vi "3D_viewer.vi"() -> ()   [LabVIEW 2015]
uses:
  <vilib>/Utility/miscctls.llb/LVRGBAColorTypeDef.ctl
  <vilib>/Utility/miscctls.llb/LV3DPointTypeDef.ctl
  <vilib>/picture/3D Picture Control/Object/Create Object (name).vi
  G_ALL.vi
  G_SEN.vi
  <vilib>/picture/3D Picture Control/NI_3D Picture Control.lvlib
panel:
  in  "obs":bool
  in  "lane":bool
  in  "map":bool
  in  "y":dbl(slide)=-32.45749613601231 scale=-1000.0..1000.0
  in  "x":dbl(slide)=53.2687651331719 scale=-1000.0..1000.0
  in  "reset camera 2":bool
  out "Translation":cluster{"X":sgl, "Y":sgl, "Z":sgl}
  out "appended path":path
  in  "reset camera":bool
  out "car obs":refnum<vi>
  out "3D Picture":refnum<vi>(3d-picture)
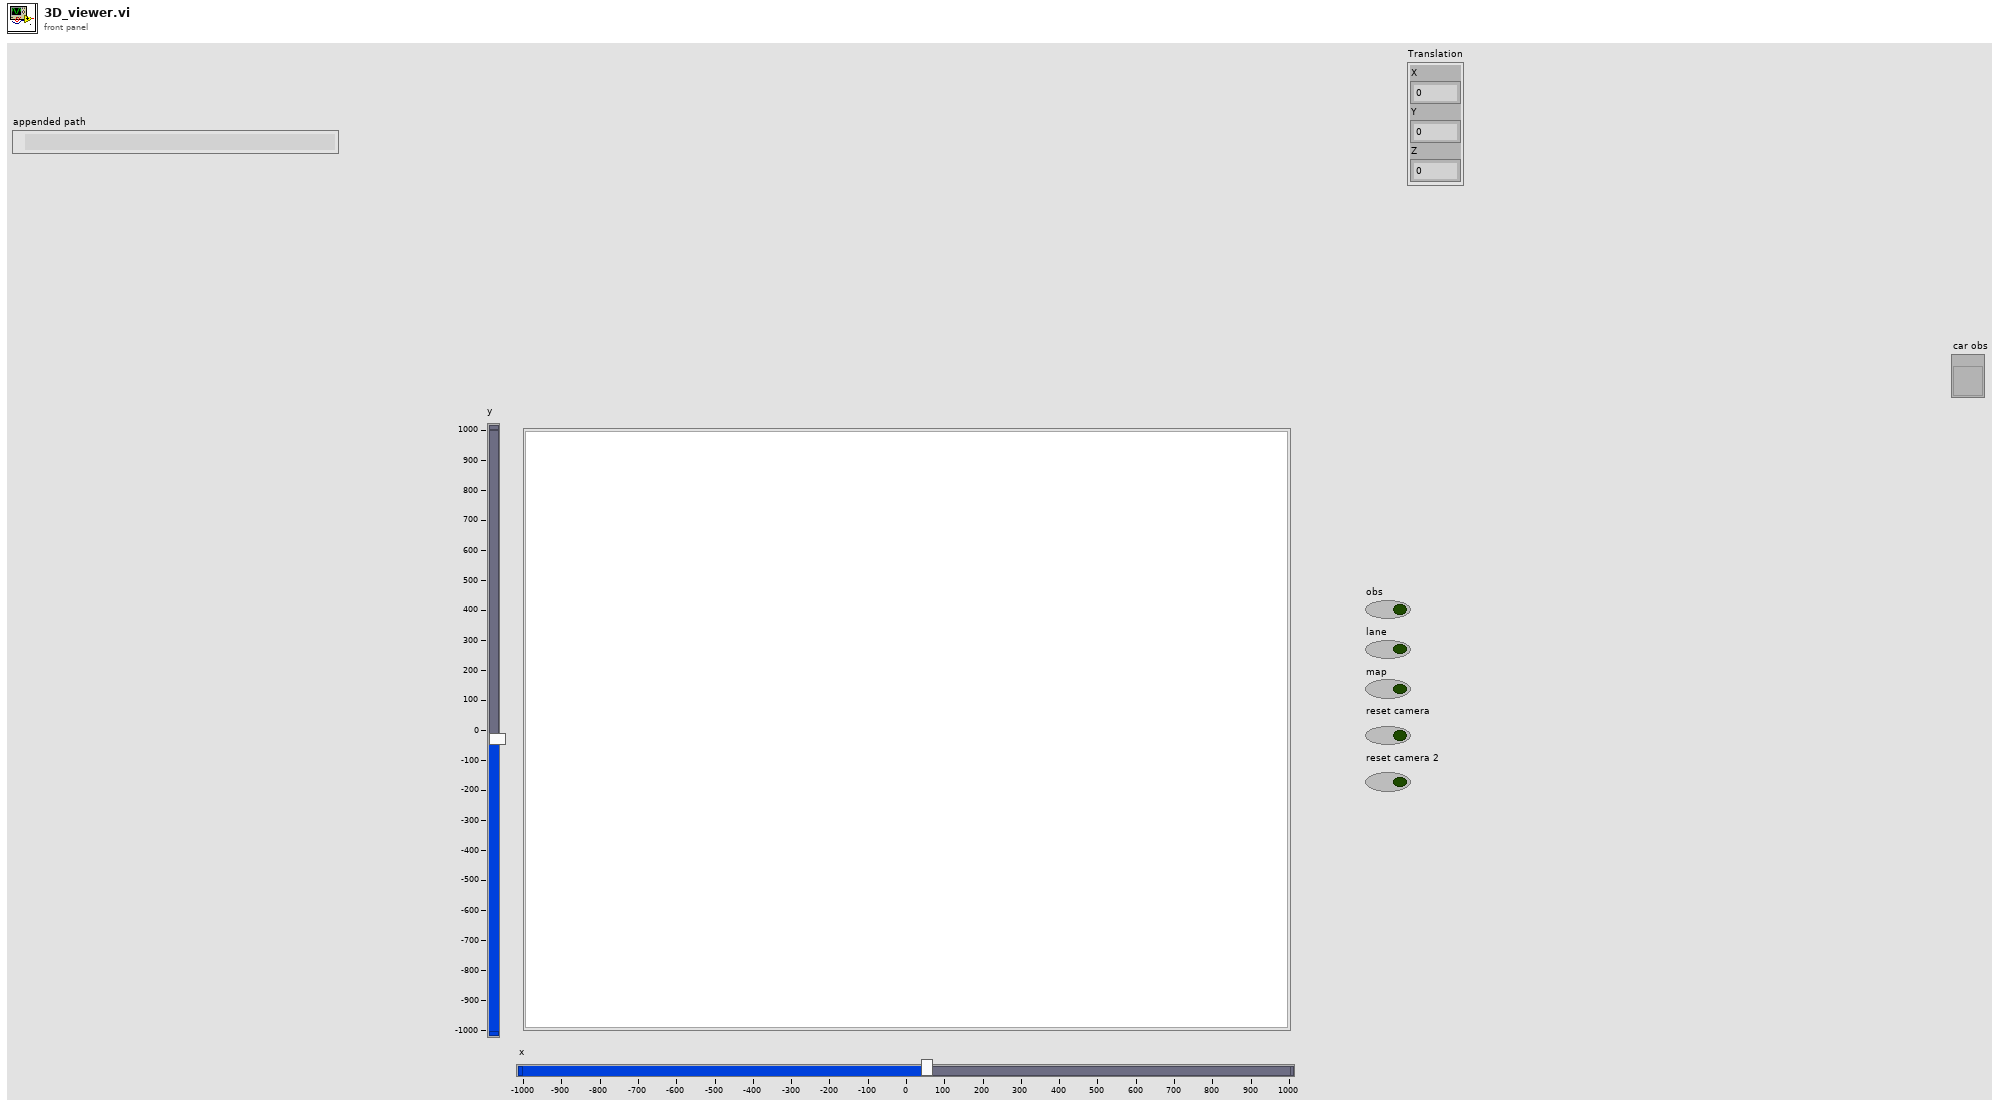
[diagram p1: front panel]
types:
  T1 = enum16{"None", "Spherical", "Flying", "Oriented"}
  T2 = cluster{"Red":sgl, "Green":sgl, "Blue":sgl, "Alpha":sgl}
  T3 = enum16{"Overall", "Per Primitive", "Per Vertex", "Binding Off"}
  T4 = typedef "LVRGBAColorTypeDef.ctl" = cluster{"Red":sgl, "Green":sgl, "Blue":sgl, "Alpha":sgl}
  T5 = enum16{"Points", "Lines", "Line Strip", "Line Loop", "Triangles", "Triangle Strip", "Triangle Fan", "Quads", "Quad Strip", "Polygon"}
  T6 = typedef "LV3DPointTypeDef.ctl" = cluster{"X":sgl, "Y":sgl, "Z":sgl}
  T7 = typedef "imagedata.ctl" = cluster{"image type":i32, "image depth":i32, "image":u8[], "mask":u8[], "colors":u32[], "Rectangle":cluster{"left":i16, "top":i16, "right":i16, "bottom":i16}}
  T8 = cluster{"left":i16, "top":i16, "right":i16, "bottom":i16}
  T9 = cluster{"left":sgl, "top":sgl, "right":sgl, "bottom":sgl}
  T10 = cluster{"Steer_input":dbl, "Steer_output":dbl, "VS_des":dbl, "VS_can":dbl, "heading":dbl, "auto":bool, "run":bool, "x":dbl, "y":dbl}
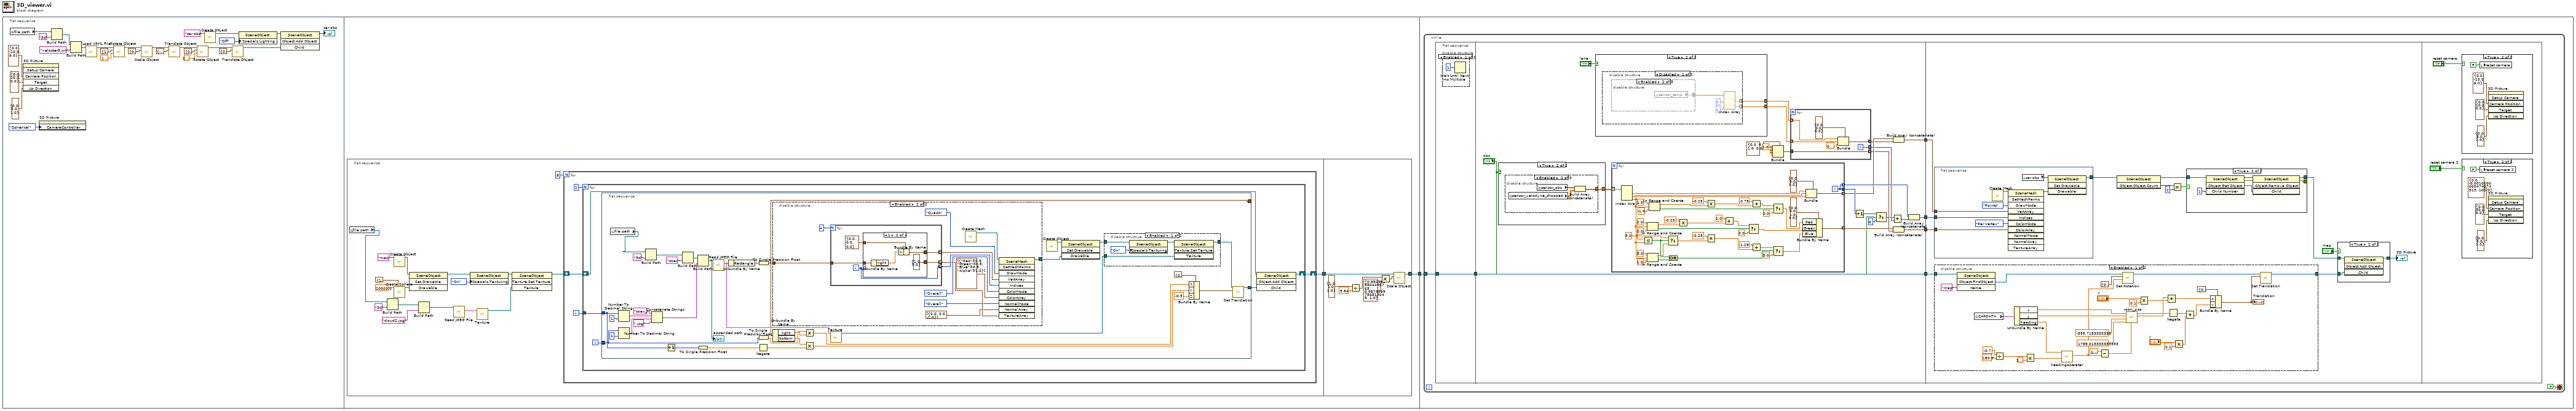
[diagram p0: block diagram]
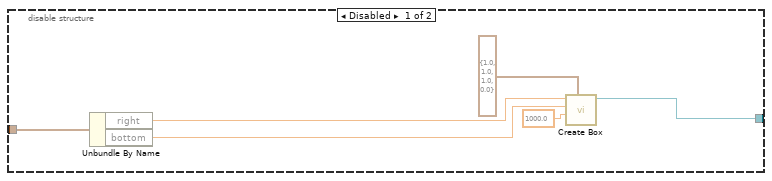
[diagram p3: hidden frame]
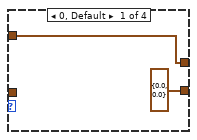
[diagram p4: hidden frame]
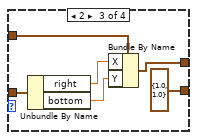
[diagram p5: hidden frame]
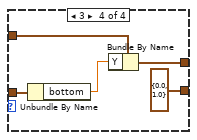
[diagram p6: hidden frame]
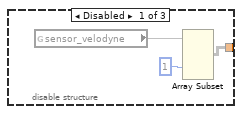
[diagram p9: hidden frame]
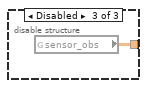
[diagram p10: hidden frame]
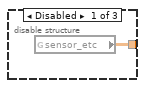
[diagram p12: hidden frame]
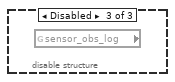
[diagram p13: hidden frame]
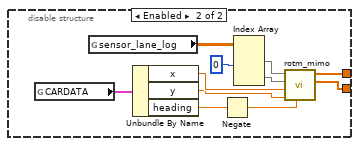
[diagram p14: hidden frame]
diagram:
  n1 = flat-sequence {
    tunnel: [w30] -> w1
    tunnel: w1 -> [w147]
    frame #0 {
      n2 = global read "G_ALL.vi" "file path"() -> (w2:path)
      n3 = invoke on="3D Picture" class="SceneGraphDisp (strict)" method="Setup Camera"("Camera Position"=cluster{"X":sgl, "Y":sgl, "Z":sgl} {"X"=0.0, "Y"=-10.0, "Z"=6.0}, "Target"=cluster{"X":sgl, "Y":sgl, "Z":sgl} {"X"=0.0, "Y"=10.0, "Z"=0.0}, "Up Direction"=cluster{"X":sgl, "Y":sgl, "Z":sgl} {"X"=0.0, "Y"=0.0, "Z"=1.0}) -> ()  [unwired: 3 in, 6 out]
      n4 = property on="3D Picture" class="SceneGraphDisp (strict)"("CameraController"=T1."Spherical" ("Camera Controller:Type")) -> ()  [unwired: 2 in, 2 out]
      n5 = Build Path(base path=w2, name or relative path="3d") -> (appended path=w25:path)
      n6 = Build Path(base path=w25, name or relative path="veloster3.wrl") -> (appended path=w27:path)
      n7 = call <vilib>:"Load VRML File.vi"("Path"=w27) -> ("Scene:Read Scene File"=w12:refnum<vi>)  [unwired: 9 in, 1 out]
      n8 = call <vilib>:"Rotate Object.vi"("Angle"=1.5707963267948966, "Axis"=cluster{"X":sgl, "Y":sgl, "Z":sgl} {"X"=1.0, "Y"=0.0, "Z"=0.0}, "Scene.Object In"=w12) -> ("Scene.Object Out"=w9:refnum<vi>)  [unwired: 7 in, 1 out]
      n9 = call <vilib>:"Scale Object.vi"("Scale"=cluster{"X":sgl, "Y":sgl, "Z":sgl} {"X"=0.055, "Y"=0.058, "Z"=0.058}, "Scene.Object In"=w9) -> ("Scene.Object Out"=w7:refnum<vi>)  [unwired: 8 in, 1 out]
      n10 = call <vilib>:"Translate Object.vi"("Translation"=cluster{"X":sgl, "Y":sgl, "Z":sgl} {"X"=-1.385, "Y"=-4.9, "Z"=-0.98}, "Scene.Object In"=w7) -> ("Scene.Object Out"=w15:refnum<vi>)  [unwired: 8 in, 1 out]
      n11 = call <vilib>:"Rotate Object.vi"("Angle"=3.141592653589793, "Axis"=cluster{"X":sgl, "Y":sgl, "Z":sgl} {"X"=0.0, "Y"=0.0, "Z"=1.0}, "Scene.Object In"=w15) -> ("Scene.Object Out"=w21:refnum<vi>)  [unwired: 7 in, 1 out]
      n12 = call-poly <vilib>:"Create Object.vi"("Name"="car obs") -> ("Scene:New Object"=w5:refnum<vi>)  [unwired: 9 in, 1 out]
      n13 = call <vilib>:"Translate Object.vi"("Translation"=cluster{"X":sgl, "Y":sgl, "Z":sgl} {"X"=0.0, "Y"=0.0, "Z"=0.2159}, "Scene.Object In"=w21) -> ("Scene.Object Out"=w22:refnum<vi>)  [unwired: 8 in, 1 out]
      n14 = property class="SceneObject"(reference=w5, "Specials.Lighting"=enum16{"Inherit Value", "Off", "On"}."Off" ("Specials:Lighting")) -> (reference out=w13:refnum<vi>)  [unwired: 1 in, 1 out]
      n15 = invoke class="SceneObject" method="Object.Add Object"(reference=w13, "Child"=w22) -> (reference out=→"car obs":refnum<vi>)  [unwired: 2 in, 3 out]
    }
    frame #1 {
      n16 = flat-sequence {
        tunnel: [w32] -> w29
        tunnel: [w145] -> w30
        tunnel: w29 -> [w146]
        frame #0 {
          n17 = global read "G_ALL.vi" "file path"() -> (w31:path)
          n18 = Build Path(base path=w31, name or relative path="3d") -> (appended path=w34:path)
          n19 = call-poly <vilib>:"Create Object.vi"("Name"="map") -> ("Scene:New Object"=w44:refnum<vi>)  [unwired: 9 in, 1 out]
          n20 = call <vilib>:"Create Sphere.vi"("Color"=T2 {"Red"=1.0, "Green"=1.0, "Blue"=1.0, "Alpha"=1.0}, "Radius"=sgl 20000.0) -> ("New Sphere Refnum"=w43:refnum<vi>)  [unwired: 8 in, 1 out]
          n21 = invoke class="SceneObject" method="Set Drawable"(reference=w44, "Drawable"=w43) -> (reference out=w42:refnum<vi>)  [unwired: 2 in, 3 out]
          n22 = Build Path(base path=w34, name or relative path="cloud2.jpg") -> (appended path=w33:path)
          n23 = call <vilib>:"Read JPEG File.vi"("path to JPEG file"=w33) -> ("image data"=w40:T7)  [unwired: 8 in, 2 out]
          n24 = property class="SceneObject"(reference=w42, "Specials.Texturing"=enum16{"Inherit Value", "Off", "On"}."On" ("Specials:Texturing")) -> (reference out=w38:refnum<vi>)  [unwired: 1 in, 1 out]
          n25 = call <vilib>:"Texture.vi"("Image"=w40) -> ("New Texture Refnum"=w39:refnum<vi>)  [unwired: 1 in, 9 out]
          n26 = invoke class="SceneObject" method="Texture.Set Texture"(reference=w38, "Texture"=w39) -> (reference out=w41:refnum<vi>)  [unwired: 2 in, 3 out]
          n27 = for {
            N: 8 -> [_]
            shift-right: [w50] -> w32
            shift-left: w41 -> [w52]
            i -> [w49]
            n28 = for {
              N: 2 -> [_]
              shift-right: [w55] -> w50
              shift-left: w52 -> [w57]
              tunnel: w49 -> [w53]
              i -> [w54]
              n29 = flat-sequence {
                tunnel: [w74] -> w56
                tunnel: w54 -> [w73]
                tunnel: w53 -> [w62]
                tunnel: [w65] -> _
                frame #0 {
                  n30 = global read "G_ALL.vi" "file path"() -> (w58:path)
                  n31 = Number To Decimal String(number=w62, width (-)=i16 1) -> (decimal integer string=w66:string)
                  n32 = Number To Decimal String(number=w73, width (-)=i16 1) -> (decimal integer string=w80:string)
                  n33 = Build Path(base path=w58, name or relative path="3d") -> (appended path=w87:path)
                  n34 = Concatenate Strings("coex_" ("string"), w66, w80, ".jpg" ("name or relative path")) -> (w78:string)
                  n35 = Increment(x=w62) -> (x+1=w61:i32)
                  n36 = Build Path(base path=w87, name or relative path="coex") -> (appended path=w85:path)
                  n37 = Build Path(base path=w85, name or relative path=w78) -> (appended path=w84:path)
                  "appended path" <- w84
                  n38 = To Single Precision Float(number=w61) -> (single precision float=w71:sgl)
                  n39 = call <vilib>:"Read JPEG File.vi"("path to JPEG file"=w84) -> ("image data"=w83:T7)  [unwired: 8 in, 2 out]
                  n40 = Unbundle By Name(w83) -> ("Rectangle"=w82:T8)
                  n41 = Negate(x=w71) -> (-x=w69:sgl)
                  n42 = To Single Precision Float(number=w82) -> (single precision float=w65:T9)
                  n43 = To Single Precision Float(number=w73) -> (single precision float=w63:sgl)
                  n44 = disable-structure shown="Enabled" {
                    disable-tunnel: [w103 w115] -> w89
                    disable-tunnel: w65 -> [w99 w110]
                    frame Disabled {
                      n45 = Unbundle By Name(w99) -> ("right"=w101:sgl, "bottom"=w100:sgl)
                      n46 = call <vilib>:"Create Box.vi"("Color"=T2 {"Red"=1.0, "Green"=1.0, "Blue"=1.0, "Alpha"=0.0}, "Length Z"=sgl 1000.0, "Length Y"=w100, "Length X"=w101) -> ("New Box Refnum"=w103:refnum<vi>)  [unwired: 6 in, 1 out]
                    }
                    frame Enabled {
                      n47 = for {
                        N: 4 -> [_]
                        tunnel: [w120] -> w112 mode=indexing
                        tunnel: [w119] -> w111 mode=indexing
                        tunnel: w110 -> [w118]
                        tunnel: [w117] -> w107 mode=indexing
                        i -> [w119]
                        n48 = case shown="1" w119 {
                          tunnel: T6 {"X"=0.0, "Y"=0.0, "Z"=0.0} ("3D Point") -> [w123 w128 w134 w139]
                          tunnel: [w123 w127 w133 w138] -> w120
                          tunnel: w118 -> [_ w126 w132 w137]
                          tunnel: [cluster{"S":sgl, "T":sgl} {"S"=0.0, "T"=0.0} cluster{"S":dbl, "T":sgl} {"S"=1.0, "T"=0.0} cluster{"S":dbl, "T":dbl} {"S"=1.0, "T"=1.0} cluster{"S":dbl, "T":dbl} {"S"=0.0, "T"=1.0}] -> w117
                          frame 0, Default {
                          }
                          frame 1 {
                            n49 = Unbundle By Name(w126) -> ("right"=w125:sgl)
                            n50 = Bundle By Name(cluster=w128, "X"=w125) -> (w127:T6)
                          }
                          frame 2 {
                            n51 = Unbundle By Name(w132) -> ("right"=w131:sgl, "bottom"=w130:sgl)
                            n52 = Bundle By Name(cluster=w134, "X"=w131, "Y"=w130) -> (w133:T6)
                          }
                          frame 3 {
                            n53 = Unbundle By Name(w137) -> ("bottom"=w136:sgl)
                            n54 = Bundle By Name(cluster=w139, "Y"=w136) -> (w138:T6)
                          }
                        }
                      }
                      n55 = call <vilib>:"Create Mesh.vi"() -> ("New Mesh Refnum"=w116:refnum<vi>)  [unwired: 10 in, 1 out]
                      n56 = invoke class="SceneMesh" method="SetMeshParms"(reference=w116, "DrawMode"=T5."Quads" ("Draw Mode"), "VertArray"=w112, "Indices"=w111, "ColorMode"=T3."Overall" ("Color Binding Mode"), "ColorArray"=T4[] [{"Red"=0.5, "Green"=0.5, "Blue"=0.5, "Alpha"=1.0}] ("Color Array"), "NormalMode"=T3."Overall" ("Normal Binding Mode"), "NormalArray"=cluster{"X":sgl, "Y":sgl, "Z":sgl}[] [{"X"=0.0, "Y"=0.0, "Z"=-1.0}], "TextureArray"=w107) -> (reference out=w115:refnum<vi>)  [unwired: 2 in, 10 out]
                    }
                  }
                  n57 = Unbundle By Name(w65) -> ("right"=w64:sgl, "bottom"=w70:sgl)
                  n58 = Multiply(x=w63, y=w64) -> (x*y=w76:sgl)
                  n59 = Multiply(x=w70, y=w69) -> (x*y=w68:sgl)
                  n60 = call <vilib>:"Texture.vi"("Image"=w83) -> ("New Texture Refnum"=w92:refnum<vi>)  [unwired: 1 in, 9 out]
                  n61 = call-poly <vilib>:"Create Object.vi"() -> ("Scene:New Object"=w90:refnum<vi>)  [unwired: 10 in, 1 out]
                  n62 = invoke class="SceneObject" method="Set Drawable"(reference=w90, "Drawable"=w89) -> (reference out=w91:refnum<vi>)  [unwired: 2 in, 3 out]
                  n63 = disable-structure shown="Enabled" {
                    disable-tunnel: w92 -> [w97 _]
                    disable-tunnel: w91 -> [w95 w98]
                    disable-tunnel: [w93 w98] -> w60
                    frame Enabled {
                      n64 = property class="SceneObject"(reference=w95, "Specials.Texturing"=enum16{"Inherit Value", "Off", "On"}."On" ("Specials:Texturing")) -> (reference out=w94:refnum<vi>)  [unwired: 1 in, 1 out]
                      n65 = invoke class="SceneObject" method="Texture.Set Texture"(reference=w94, "Texture"=w97) -> (reference out=w93:refnum<vi>)  [unwired: 2 in, 3 out]
                    }
                    frame Disabled {
                    }
                  }
                  n66 = Bundle By Name(cluster=cluster{"X":sgl, "Y":sgl, "Z":sgl} {"X"=0.0, "Y"=0.0, "Z"=0.0} ("Translation"), "X"=w76, "Y"=w68, "Z"=sgl -0.5) -> (w75:cluster{"X":sgl, "Y":sgl, "Z":sgl})
                  n67 = call <vilib>:"Set Translation.vi"("Translation"=w75, "Scene Object"=w60) -> ("Translated Object"=w74:refnum<vi>)  [unwired: 8 in, 1 out]
                }
              }
              n68 = invoke class="SceneObject" method="Object.Add Object"(reference=w57, "Child"=w56) -> (reference out=w55:refnum<vi>)  [unwired: 2 in, 3 out]
            }
          }
        }
        frame #1 {
          n69 = Divide(x=cluster{"X":sgl, "Y":sgl, "Z":sgl} {"X"=1.0, "Y"=1.0, "Z"=1.0} ("Scale"), y=sgl 5.85 ("Y")) -> (x/y=w142:cluster{"X":sgl, "Y":sgl, "Z":sgl})
          n70 = Multiply(x=w142, y=cluster{"X":sgl, "Y":sgl, "Z":sgl} {"X"=0.983, "Y"=0.988, "Z"=1.0} ("Scale")) -> (x*y=w140:cluster{"X":sgl, "Y":sgl, "Z":sgl})
          n71 = call <vilib>:"Scale Object.vi"("Scale"=w140, "Scene.Object In"=w146) -> ("Scene.Object Out"=w145:refnum<vi>)  [unwired: 8 in, 1 out]
        }
      }
    }
    frame #2 {
      n72 = while {
        tunnel: w147 -> [w148]
        stop <- FALSE stop-if-true
        n73 = flat-sequence {
          tunnel: [w155] -> w149
          tunnel: w148 -> [w155]
          tunnel: [w165] -> w153
          tunnel: [w168] -> w152
          tunnel: [w162] -> w151
          tunnel: [w178] -> w150
          tunnel: w149 -> [w178]
          tunnel: w151 -> [w269]
          tunnel: w152 -> [w268]
          tunnel: w153 -> [w270]
          tunnel: w150 -> [w267]
          frame #0 {
            n74 = disable-structure shown="Enabled" {
              frame Enabled {
                n75 = Wait Until Next ms Multiple(millisecond multiple=u32 1) -> ()  [unwired: 1 out]
              }
              frame Disabled {
              }
            }
          }
          frame #1 {
            w177 = sgl 1.0 ("Red")
            n76 = case shown="True" "obs" {
              tunnel: [_ w180] -> w179
              frame False {
              }
              frame True {
                n77 = disable-structure shown="Enabled" {
                  disable-tunnel: [w181 w184 w187] -> w180
                  frame Disabled {
                    n78 = global read "G_SEN.vi" "sensor_velodyne"() -> (w183)
                    n79 = Array Subset(array=w183, index (col)=1 ("index")) -> (w181:void[][])  [unwired: 3 in]
                  }
                  frame Enabled {
                    n80 = global read "G_SEN.vi" "sensor_velodyne_chopped"() -> (w185:dbl[][])
                    n81 = global read "G_SEN.vi" "sensor_obs"() -> (w186:dbl[][])
                    n82 = Build Array (concatenate)(w186, w185) -> (w184:dbl[][])
                  }
                  frame Disabled {
                    n83 = global read "G_SEN.vi" "sensor_obs"() -> (w187:dbl[][])
                  }
                }
              }
            }
            n84 = case shown="True" "lane" {
              tunnel: [_ w189] -> w174
              tunnel: [_ w188] -> w173
              frame False {
              }
              frame True {
                n85 = disable-structure shown="Disabled" {
                  disable-tunnel: [w194 w198] -> w188
                  disable-tunnel: [w193 w199] -> w189
                  frame Disabled {
                    n86 = disable-structure shown="Enabled" {
                      disable-tunnel: [w195 w196 _] -> w192
                      frame Disabled {
                        n87 = global read "G_SEN.vi" "sensor_etc"() -> (w195:dbl[][])
                      }
                      frame Enabled {
                        n88 = global read "G_SEN.vi" "sensor_temp"() -> (w196)
                      }
                      frame Disabled {
                        n89 = global read "G_SEN.vi" "sensor_obs_log"() -> ()  [unwired: 1 out]
                      }
                    }
                    n90 = Index Array(array=w192, index (col) #1=0 ("disabled index (col)"), index (col) #2=1 ("index (col)")) -> (element #1=w193:dbl[], element #2=w194:dbl[])  [unwired: 2 in]
                  }
                  frame Enabled {
                    n91 = global read "G_ALL.vi" "CARDATA"() -> (w197:T10)
                    n92 = global read "G_SEN.vi" "sensor_lane_log"() -> (w206:dbl[][])
                    n93 = Unbundle By Name(w197) -> ("x"=w205:dbl, "y"=w204:dbl, "heading"=w203:dbl)
                    n94 = Negate(x=w203) -> (-x=w202:dbl)
                    n95 = Index Array(array=w206, index (col) #1=0 ("disabled index (col)")) -> (element #1=w201:dbl[], element #2=w200:dbl[])  [unwired: 3 in]
                    n96 = call "rotm_mimo.vi"("angle[rad]"=w202, "y0"=w204, "x0"=w205, "y"=w200, "x"=w201) -> ("Y"=w198:dbl[], "X"=w199:dbl[])  [unwired: 3 in, 2 out]
                  }
                }
              }
            }
            n97 = for {
              tunnel: w179 -> [w257] mode=indexing
              tunnel: [w253] -> w167 mode=indexing
              tunnel: [w222] -> w169 mode=indexing
              tunnel: [w248] -> w164 mode=indexing
              tunnel: [w222] -> w171
              i -> [w222]
              w220 = 3.0 ("upper limit")
              n98 = Index Array(array=w257) -> (element #1=w255:dbl, element #2=w254:dbl, element #3=w221:dbl)  [unwired: 3 in]
              n99 = Less Or Equal?(x=w220, y=w221) -> (x <= y?=w215:bool)
              n100 = In Range and Coerce(upper limit=2.0, x=w221, lower limit=0.0) -> (coerced(x)=w246:dbl, In Range?=w227:bool)
              n101 = In Range and Coerce(upper limit=3.0, x=w221, lower limit=1.0) -> (coerced(x)=w219:dbl, In Range?=w217:bool)
              n102 = In Range and Coerce(upper limit=1.0, x=w221, lower limit=-1.0) -> (coerced(x)=w233:dbl, In Range?=w234:bool)
              n103 = Select(t=w220, s=w215, f=w219) -> (s? t:f=w218:dbl)
              n104 = Or(x=w215, y=w217) -> (x .or. y?=w216:bool)
              n105 = Multiply(x=-0.25, y=w246) -> (x*y=w236:dbl)
              n106 = Multiply(x=-0.25, y=w233) -> (x*y=w240:dbl)
              n107 = Multiply(x=-0.25, y=w218) -> (x*y=w238:dbl)
              n108 = Add(x=1.0, y=w236) -> (x+y=w228:dbl)
              n109 = Select(t=w228, s=w227, f=0.0) -> (s? t:f=w226:dbl)
              n110 = Add(x=0.75, y=w240) -> (x+y=w232:dbl)
              n111 = Add(x=1.25, y=w238) -> (x+y=w224:dbl)
              n112 = Select(t=w232, s=w234, f=0.0) -> (s? t:f=w230:dbl)
              n113 = Select(t=w224, s=w216, f=0.0) -> (s? t:f=w223:dbl)
              n114 = Bundle By Name(cluster=T4 {"Red"=0.0, "Green"=0.0, "Blue"=1.0, "Alpha"=0.0} ("Color"), "Red"=w230, "Green"=w226, "Blue"=w223) -> (w248:T4)
              n115 = Bundle(cluster=T6 {"X"=0.0, "Y"=0.0, "Z"=0.0} ("3D Point"), "X"=w255, "Y"=w254, "Z"=w221) -> (w253:T6)
            }
            n116 = Bundle(cluster=T4 {"Red"=0.0, "Green"=0.0, "Blue"=1.0, "Alpha"=0.0} ("Color"), "Red"=w177, "Green"=w177, "Blue"=w177, "Alpha"=w177) -> (w175:T4)
            n117 = for {
              tunnel: [w214] -> w163 mode=indexing
              tunnel: w175 -> [w214]
              tunnel: [w208] -> w170 mode=indexing
              tunnel: w174 -> [w212] mode=indexing
              tunnel: w173 -> [w211] mode=indexing
              tunnel: [w209] -> w166 mode=indexing
              i -> [w208]
              n118 = Bundle(cluster=T6 {"X"=0.0, "Y"=0.0, "Z"=0.0} ("3D Point"), "X"=w212, "Y"=w211, "Z"=sgl 0.1) -> (w209:T6)
            }
            n119 = Increment(x=w171) -> (x+1=w159:i32)
            n120 = Select(t=w159, s="obs", f=0) -> (s? t:f=w158:i32)
            n121 = Add(x=w158, y=w170) -> (x+y=w172:i32[])
            n122 = Build Array (concatenate)(w167, w166) -> (w165:T6[])
            n123 = Build Array (concatenate)(w164, w163) -> (w162:T4[])
            n124 = Build Array (concatenate)(w169, w172) -> (w168:i32[])
          }
          frame #2 {
            n125 = flat-sequence {
              tunnel: w270 -> [w324]
              tunnel: w269 -> [w323]
              tunnel: w268 -> [w322]
              tunnel: [w317] -> w263
              frame #0 {
                n126 = call <vilib>:"Create Mesh.vi"() -> ("New Mesh Refnum"=w319:refnum<vi>)  [unwired: 10 in, 1 out]
                n127 = invoke class="SceneMesh" method="SetMeshParms"(reference=w319, "DrawMode"=T5."Points" ("Draw Mode"), "VertArray"=w324, "Indices"=w322, "ColorMode"=T3."Per Vertex" ("Color Binding Mode"), "ColorArray"=w323) -> (reference out=w318:refnum<vi>)  [unwired: 5 in, 10 out]
                n128 = local read "car obs"() -> (w325:refnum<vi>)
                n129 = invoke class="SceneObject" method="Set Drawable"(reference=w325, "Drawable"=w318) -> (reference out=w317:refnum<vi>)  [unwired: 2 in, 3 out]
              }
            }
            n130 = disable-structure shown="Enabled" {
              disable-tunnel: w267 -> [w302 w304]
              disable-tunnel: [w272 w304] -> w265
              frame Enabled {
                n131 = invoke class="SceneObject" method="Object.FindObject"(reference=w302, "Name"="map") -> ("FindObject"=w298:refnum<vi>)  [unwired: 2 in, 3 out]
                n132 = global read "G_ALL.vi" "CARDATA"() -> (w271:T10)
                n133 = Divide(x=-0.7 ("Numeric"), y=180.0) -> (x/y=w285:dbl)
                n134 = Unbundle By Name(w271) -> ("x"=w293:dbl, "y"=w292:dbl, "heading"=w289:dbl)
                n135 = Multiply(x=w285, y=3.141592653589793) -> (x*y=w283:dbl)
                n136 = call "headingoperater.vi"("h1"=w283, "h2"=w289) -> ("h2-h1"=w288:dbl)  [unwired: 8 in, 1 out]
                n137 = Subtract(x=1.5707963267948966, y=w288) -> (x-y=w296:dbl)
                n138 = call <vilib>:"Set Rotation.vi"("Angle"=w288, "Axis"=cluster{"X":sgl, "Y":sgl, "Z":sgl} {"X"=0.0, "Y"=0.0, "Z"=1.0}, "Scene Object"=w298) -> ("Rotated Scene Object"=w300:refnum<vi>)  [unwired: 7 in, 1 out]
                n139 = call "rotm_siso.vi"("angle[rad]"=w296, "y0"=1789.013333333333, "x0"=-595.7153333333, "y"=w292, "x"=w293) -> ("y'"=w282:dbl, "x'"=w291:dbl)  [unwired: 5 in]
                n140 = Multiply(x="x", y=0.1) -> (x*y=w279:dbl)
                n141 = Add(x=w282, y=w279) -> (x+y=w278:dbl)
                n142 = Negate(x=w291) -> (-x=w277:dbl)
                n143 = Multiply(x="y", y=0.1) -> (x*y=w273:dbl)
                n144 = Add(x=w277, y=w273) -> (x+y=w276:dbl)
                n145 = Bundle By Name(cluster=cluster{"X":sgl, "Y":sgl, "Z":sgl} {"X"=0.0, "Y"=0.0, "Z"=0.0} ("Translation"), "X"=w278, "Y"=w276) -> (w299:cluster{"X":sgl, "Y":sgl, "Z":sgl})
                "Translation" <- w299
                n146 = call <vilib>:"Set Translation.vi"("Translation"=w299, "Scene Object"=w300) -> ("Translated Object"=w272:refnum<vi>)  [unwired: 8 in, 1 out]
              }
              frame Disabled {
              }
            }
            n147 = invoke class="SceneObject" method="Object.Object Count"(reference=w263) -> (reference out=w259:refnum<vi>, "Child Count"=w262:i32)  [unwired: 2 in, 1 out]
            n148 = Equal?(x=w262, y=2) -> (x = y?=w260:bool)
            n149 = case shown="True" w260 {
              tunnel: [w305 w312] -> w266
              tunnel: [_ w308] -> _
              tunnel: w259 -> [w305 w307]
              frame False {
              }
              frame True {
                n150 = invoke class="SceneObject" method="Object.Get Object"(reference=w307, "Child Number"=1 ("index")) -> (reference out=w311:refnum<vi>, error out=w309:errorcluster, "Get Child"=w310:refnum<vi>)  [unwired: 2 in, 1 out]
                n151 = invoke class="SceneObject" method="Object.Remove Object"(reference=w311, error in=w309, "Child"=w310) -> (reference out=w312:refnum<vi>, error out=w308:errorcluster)  [unwired: 1 in, 2 out]
              }
            }
            n152 = case shown="True" "map" {
              tunnel: w266 -> [w313 w316]
              tunnel: [w313 w315] -> w258
              tunnel: w265 -> [_ w314]
              frame False {
              }
              frame True {
                n153 = invoke class="SceneObject" method="Object.Add Object"(reference=w316, "Child"=w314) -> (reference out=w315:refnum<vi>)  [unwired: 2 in, 3 out]
              }
            }
            "3D Picture" <- w258
          }
          frame #3 {
            n154 = case shown="True" "reset camera" {
              frame False {
              }
              frame True {
                n155 = local write "reset camera"(FALSE ("reset camera")) -> ()
                n156 = invoke on="3D Picture" class="SceneGraphDisp (strict)" method="Setup Camera"("Camera Position"=cluster{"X":sgl, "Y":sgl, "Z":sgl} {"X"=0.0, "Y"=-10.0, "Z"=6.0}, "Target"=cluster{"X":sgl, "Y":sgl, "Z":sgl} {"X"=0.0, "Y"=10.0, "Z"=0.0}, "Up Direction"=cluster{"X":sgl, "Y":sgl, "Z":sgl} {"X"=0.0, "Y"=0.0, "Z"=1.0}) -> ()  [unwired: 3 in, 6 out]
              }
            }
            n157 = case shown="True" "reset camera 2" {
              frame False {
              }
              frame True {
                n158 = local write "reset camera 2"(FALSE ("reset camera")) -> ()
                n159 = invoke on="3D Picture" class="SceneGraphDisp (strict)" method="Setup Camera"("Camera Position"=cluster{"X":sgl, "Y":sgl, "Z":sgl} {"X"=0.0, "Y"=-0.001, "Z"=100.0}, "Target"=cluster{"X":sgl, "Y":sgl, "Z":sgl} {"X"=0.0, "Y"=30.0, "Z"=0.0}, "Up Direction"=cluster{"X":sgl, "Y":sgl, "Z":sgl} {"X"=0.0, "Y"=0.0, "Z"=1.0}) -> ()  [unwired: 3 in, 6 out]
              }
            }
          }
        }
      }
    }
  }
